vi "Convert LabVIEW Font Size to px.vi"(11 "LabVIEW Font Size":u32) -> (3 "px Font Size":i32)   [LabVIEW 2017, in "Front Panel Publisher.lvlib" / "String.lvclass"]
uses:
  Front Panel Objects/String_class/String.lvclass
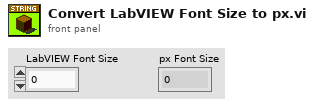
[diagram p1: front panel]
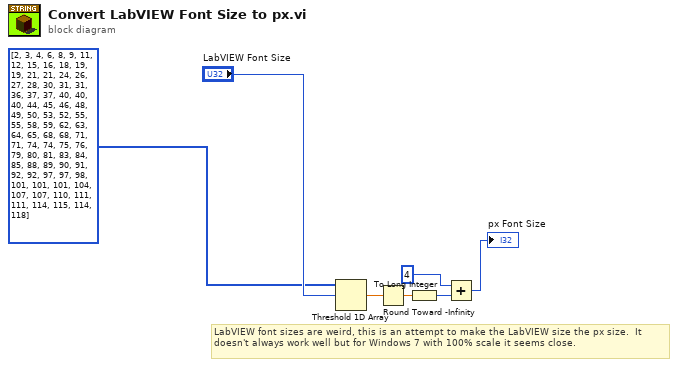
[diagram p0: block diagram]
diagram:
  # "LabVIEW font sizes are weird, this is an attempt to make the LabVIEW size the px size.  It doesn't always work well but for Windows 7 with 100% scale it seems close."
  n1 = Threshold 1D Array(2:"LabVIEW Font Size", 3:i32[] [2, 3, 4, 6, 8, 9, 11, 12, 15, 16, 18, 19, 19, 21, 21, 24, 26, 27, 28, 30, 31, 31, 36, 37, 37, 40, 40, 40, 44, 45, 46, 48, 49, 50, 53, 52, 55, 55, 58, 59, 62, 63, 64, 65, 68, 68, 71, 71, 74, 74, 75, 76, 79, 80, 81, 83, 84, 85, 88, 89, 90, 91, 92, 92, 97, 97, 98, 101, 101, 101, 104, 107, 107, 110, 111, 111, 114, 115, 114, 118] ("Array")) -> (0:w2:dbl)  [unwired: 1 in]
  n2 = Round Toward -Infinity(1:w2) -> (0:w4:dbl)
  n3 = To Long Integer(number=w4) -> (32bit integer=w5:i32)
  n4 = Add(x=4, y=w5) -> (x+y=→"px Font Size":i32)
